vi "Mock Call.vi"(8 "error in (no error)":errorcluster, 10 "Control Values":cluster{"Name":string, "Variant Data":variant}[](array[cluster]), 11 "Mock In":refnum<class "Pure Mock.lvclass">) -> (0 "error out":errorcluster, 3 "Mock Out":refnum<class "Pure Mock.lvclass">)   [LabVIEW 2020, in "Pure Mock.lvclass"]
uses:
  Pure Mock.lvclass
  Pure Mock.lvclass/Pure Mock.ctl
  Parametric VI Call/Parametric VI Call.lvclass
  C:/git/astemes-lmock/source/Core/VI Call/VI Call.lvclass
  Core/Expectation/Expectation.lvclass
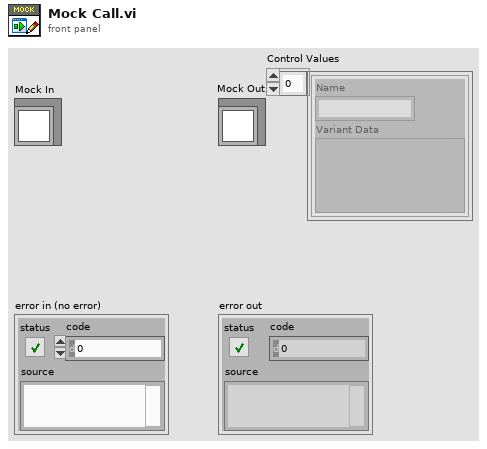
[diagram p1: front panel]
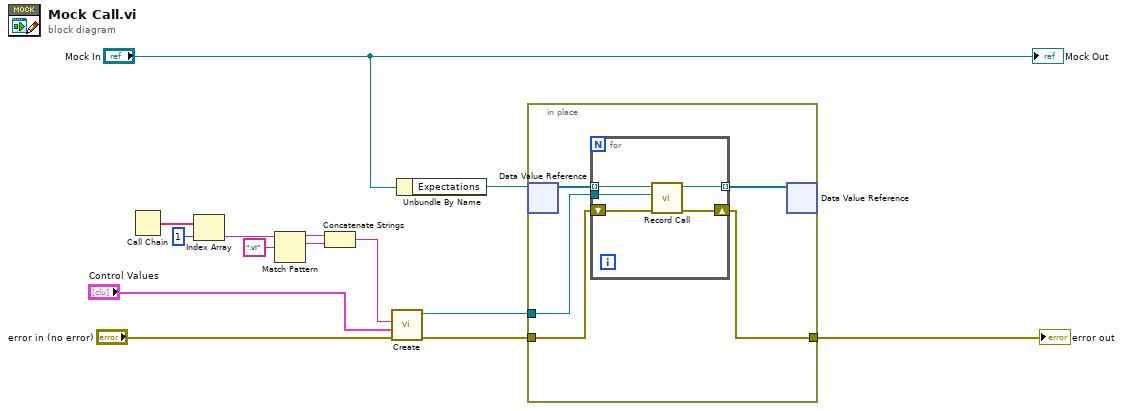
[diagram p0: block diagram]
diagram:
  n1 = Call Chain() -> (call chain=w7:string[])
  n2 = Index Array(array=w7, index=1) -> (element=w2:string)
  n3 = Match Pattern(string=w2, regular expression=".vi") -> (before substring=w4:string, match substring=w3:string)  [unwired: 1 in, 2 out]
  n4 = Concatenate Strings(w4, w3) -> (w1:string)
  n5 = call "Create.vi"("error in (no error)"="error in (no error)", "Control Values"="Control Values", "VI Name"=w1) -> ("error out"=w10:errorcluster, "Parametric VI Call Out"=w9:refnum<class "Parametric VI Call.lvclass">)  [unwired: 7 in]
  n6 = Unbundle By Name("Mock In") -> ("Expectations"=w14:refnum<data-value>)
  n7 = in-place {
    in-place-border: [w19] -> w12
    in-place-border: w10 -> [w18]
    in-place-border: w9 -> [w15]
    n8 = in-place-dvr #1(w14) -> (w17:refnum<class "Expectation.lvclass">[])  [unwired: 1 out]
    n9 = for {
      tunnel: w17 -> [w24] mode=indexing
      tunnel: [w23] -> w16 mode=indexing
      shift-right: [w22] -> w19
      shift-left: w18 -> [w21]
      tunnel: w15 -> [w20]
      n10 = call-dynamic "Record Call.vi"("error in (no error)"=w21, "VI Call"=w20, "Expectation in"=w24) -> ("error out"=w22:errorcluster, "Expectation out"=w23:refnum<class "Expectation.lvclass">)  [unwired: 7 in]
    }
    n11 = in-place-dvr #1(w16) -> ()  [unwired: 2 out]
  }
  "error out" <- w12
  "Mock Out" <- "Mock In"
